vi "oax_Generate Phase Modulated Signal (Block).vi"(5 "acc transition ratio":dbl=0.05, 6 "init phase":dbl, 7 "fs":dbl, 8 "phase":dbl, 9 "order":dbl, 10 "passed samples in":cluster{"pre":dbl, "mid":dbl, "post":dbl}, 11 "current speed positions":T1(array[cluster])) -> (2 "passed samples in":cluster{"pre":dbl, "mid":dbl, "post":dbl}, 3 "y":dbl[](array[numeric]), 4 "final phase":dbl)   [LabVIEW 2017]
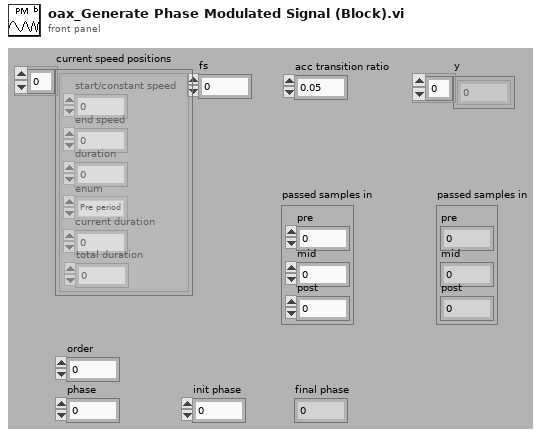
[diagram p1: front panel]
types:
  T1 = cluster{"start/constant speed":dbl, "end speed":dbl, "duration":dbl, "enum":enum16{"Pre period", "Middle period", "Post period"}, "current duration":dbl, "total duration":dbl}[]
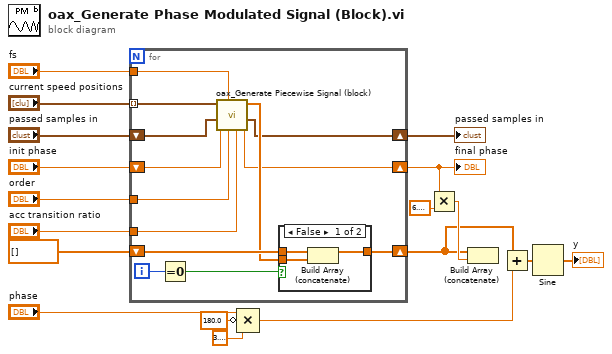
[diagram p0: block diagram]
diagram:
  n1 = for {
    tunnel: "order" -> [w31]
    tunnel: "fs" -> [w30]
    shift-right: [w28] -> w4
    shift-left: dbl[] [] ("speed 2") -> [w29]
    shift-right: [w26] -> w8
    shift-left: "init phase" -> [w25]
    tunnel: "current speed positions" -> [w24] mode=indexing
    tunnel: "acc transition ratio" -> [w23]
    shift-right: [w20] -> w1
    shift-left: "passed samples in" -> [w19]
    i -> [w21]
    n2 = Equal To 0?(x=w21) -> (x = 0?=w22:bool)
    n3 = call <vilib>:"oax_Generate Piecewise Signal (block).vi"("acc transition ratio"=w23, "order"=w31, "fs"=w30, "init phase"=w25, "passed samples in"=w19, "position"=w24) -> ("final phase"=w26:dbl, "passed samples out"=w20:cluster{"pre":dbl, "mid":dbl, "post":dbl}, "phase out"=w27:dbl[])  [unwired: 3 in]
    n4 = case shown="False" w22 {
      tunnel: w27 -> [w33 w35]
      tunnel: w29 -> [w34 _]
      tunnel: [w32 w35] -> w28
      frame False {
        n5 = Build Array (concatenate)(w34, w33) -> (w32:dbl[])
      }
      frame True {
      }
    }
  }
  "final phase" <- w8
  "passed samples in" <- w1
  n6 = Compound Arithmetic op=MULTIPLY("phase", invert 180.0 ("value"), 3.141592653589793) -> (w10:dbl)
  n7 = Multiply(x=w8, y=6.283185307179586) -> (x*y=w7:dbl)
  n8 = Build Array (concatenate)(w4, w7) -> ()  [unwired: 1 out]
  n9 = Add(x=w4, y=w10) -> (x+y=w18:dbl[])
  n10 = Sine(x=w18) -> (sin(x)=→"y":dbl[])
